vi "FTW-Client-Construct.vi"(5 "Server Address":string, 11 "error in":errorcluster) -> (4 "FTW-Client Out":refnum<class "FTW-Client.lvclass">, 15 "error out":errorcluster)   [LabVIEW 2013, in "FTW-Client.lvclass"]
uses:
  FTW-Client.lvclass
  Ether/FTW-Ether-EndpointType.ctl
  Endpoint/FTW-Endpoint.lvclass
  FTW-Client.lvclass/FTW-Client.ctl
  Ether/FTW-Ether.lvclass
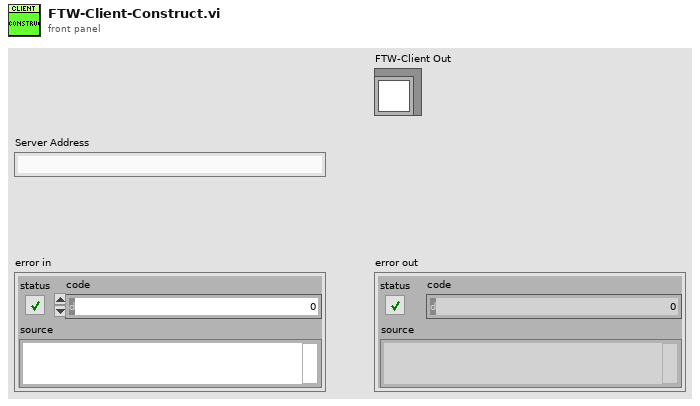
[diagram p1: front panel]
types:
  T1 = typedef "FTW-Ether.lvclass/FTW-Ether-EndpointType.ctl" = enum16{"Server", "Client", "Publisher", "Subscriber"}
  T2 = typedef "FTW-Ether.lvclass/FTW-Ether-MessageTransportScheme.ctl" = enum16{"LabVIEW Queues (lvq://)", "TCP (tcp://)", "LabVIEW Network Streams (lvns://)"}
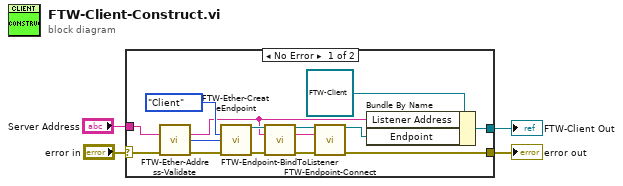
[diagram p0: block diagram]
diagram:
  n1 = case shown="No Error" "error in" {
    selector: "error in" -> [w17 w20]
    tunnel: [w7 w20] -> w2
    tunnel: [w18 _] -> w4
    tunnel: "Server Address" -> [w9 _]
    frame No Error {
      n2 = call "FTW-Ether-Address-Validate.vi"("Address"=w9, "error in"=w17) -> ("Sanitized Address"=w5:string, "Message Transport Scheme"=w10:T2, "error out"=w14:errorcluster)  [unwired: 11 in]
      n3 = call "FTW-Ether-CreateEndpoint.vi"("Endpoint Type"=FTW-Ether-EndpointType."Client", "Message Transport Scheme"=w10, "error in"=w14) -> ("FTW Endpoint"=w12:refnum<class "FTW-Endpoint.lvclass">, "error out"=w13:errorcluster)  [unwired: 11 in]
      n4 = call-dynamic "FTW-Endpoint-BindToListener.vi"("FTW-Endpoint In"=w12, "Address"=w5, "error in"=w13) -> ("FTW-Endpoint Out"=w16:refnum<class "FTW-Endpoint.lvclass">, "Actual Address"=w6:string, "error out"=w8:errorcluster)  [unwired: 10 in]
      n5 = call-dynamic "FTW-Endpoint-Connect.vi"("FTW Endpoint"=w16, "Endpoint Address"=w6, "error in"=w8) -> ("FTW Endpoint out"=w15:refnum<class "FTW-Endpoint.lvclass">, "error out"=w7:errorcluster)  [unwired: 11 in]
      n6 = Bundle By Name(cluster=refnum<class "FTW-Client.lvclass"> refnum ("LVmsg_Client in"), "Listener Address"=w5, "Endpoint"=w15) -> (w18:refnum<class "FTW-Client.lvclass">)
    }
    frame Error {
    }
  }
  "FTW-Client Out" <- w4
  "error out" <- w2
